vi "UDPHeader.vi"(11 "String in":string) -> (2 "String out":string, 3 "UDP header":T1)   [LabVIEW 2017]
panel:
  out "reversed":string
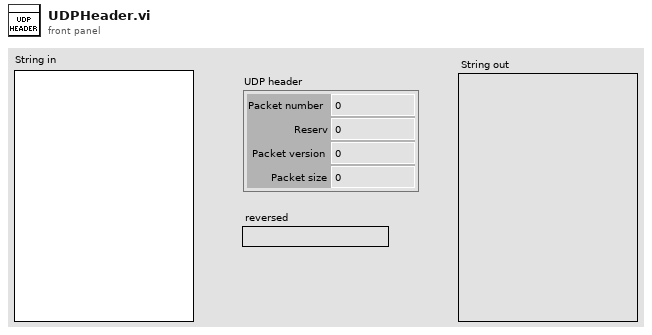
[diagram p1: front panel]
types:
  T1 = cluster{"Packet number":u32, "Reserv":u8, "Packet version":u8, "Packet size":u16}
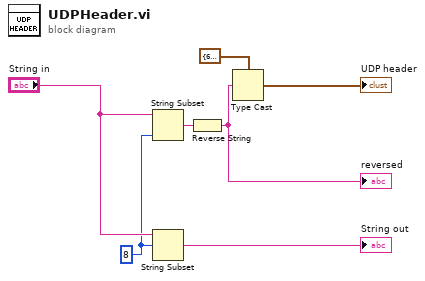
[diagram p0: block diagram]
diagram:
  w1 = 8 ("offset (0)")
  n1 = String Subset(string="String in", length (rest)=w1) -> (substring=w7:string)  [unwired: 1 in]
  n2 = String Subset(string="String in", offset (0)=w1) -> (substring=→"String out":string)  [unwired: 1 in]
  n3 = Reverse String(1:w7) -> (0:w5:string)
  "reversed" <- w5
  n4 = Type Cast(type=T1 {"Packet number"=601489409, "Reserv"=0, "Packet version"=0, "Packet size"=6400} ("*(type *) &x"), x=w5) -> (*(type *) &x=→"UDP header":T1)
